vi "Parse Transfer.vi"(8 "error in (no error)":errorcluster, 9 "inline?":bool, 10 "Transfer":refnum<class "Transfer.lvclass">, 11 "Buffer Converter in":refnum<class "Buffer Converter.lvclass">) -> (0 "error out":errorcluster, 3 "Buffer Converter out":refnum<class "Buffer Converter.lvclass">)   [LabVIEW 2017, in "DSF Core.lvlib" / "Buffer Converter.lvclass"]
uses:
  Buffer Converter.lvclass
  Transfer/Transfer.lvclass
  Buffer Converter.lvclass/Buffer Converter.ctl
  Transfer/Transfer.lvclass/Transfer.ctl
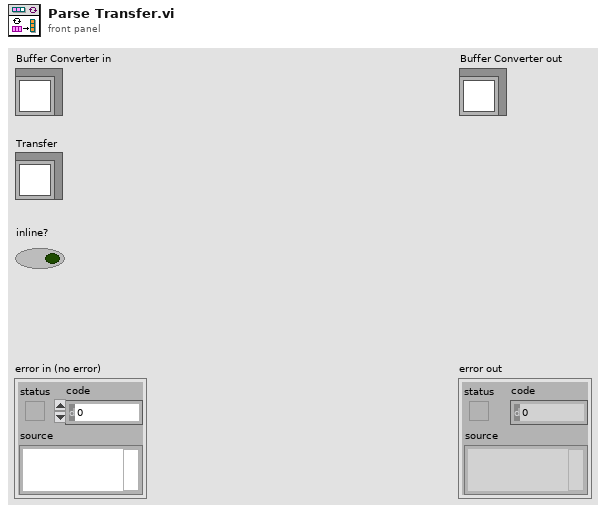
[diagram p1: front panel]
types:
  T1 = typedef "DSF Core.lvlib/Buffer Converter.lvclass/Type Conversion Descriptor.ctl" = cluster{"conversions":T2[]}
  T2 = typedef "DSF Core.lvlib/Buffer Converter.lvclass/Type Conversion.ctl" = cluster{"unconverted descriptor":T3, "converted descriptor":T3, "channel count":u64}
  T3 = typedef "DSF Core.lvlib/Buffer.lvclass/Channel Descriptor.ctl" = cluster{"buffer offset":u64, "data type":T4}
  T4 = typedef "DSF Core.lvlib/DSF Data Type.ctl" = enum8{"Bool", "SGL", "DBL", "I8", "I16", "I32", "I64", "U8", "U16", "U32", "U64"}
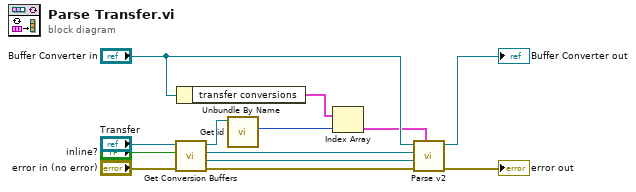
[diagram p0: block diagram]
diagram:
  n1 = call "Get Conversion Buffers.vi"("error in (no error)"="error in (no error)", "inline?"="inline?", "Transfer in"="Transfer") -> ("error out"=w9:errorcluster, "converted Buffer"=w8:refnum<class "Buffer.lvclass">, "unconverted Buffer"=w10:refnum<class "Buffer.lvclass">, "Transfer out"=w13:refnum<class "Transfer.lvclass">)  [unwired: 5 in]
  n2 = Unbundle By Name("Buffer Converter in") -> ("transfer conversions"=w12:T1[])
  n3 = call "Get id.vi"("Transfer in"=w13) -> ("id"=w11:i32)  [unwired: 9 in, 1 out]
  n4 = Index Array(array=w12, index=w11) -> (element=w1:T1)
  n5 = call-dynamic "Parse v2.vi"("conversion descriptor"=w1, "error in (no error)"=w9, "converted Buffer"=w8, "unconverted Buffer"=w10, "Buffer Converter in"="Buffer Converter in") -> ("error out"=→"error out":errorcluster, "Buffer Converter out"=→"Buffer Converter out":refnum<class "Buffer Converter.lvclass">)  [unwired: 5 in]
